vi "GetInvaderBlockEdges.vi"(11 "InvaderPosArray":T2) -> (3 "output cluster":T1)   [LabVIEW 2022 SP3]
uses:
  InvaderPositionArray.ctl
  move_dir_lr.ctl
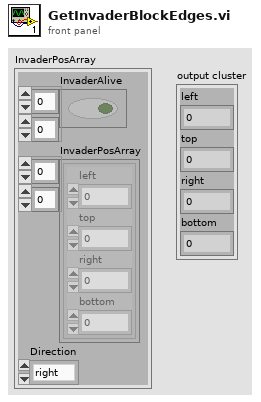
[diagram p1: front panel]
types:
  T1 = cluster{"left":i16, "top":i16, "right":i16, "bottom":i16}
  T2 = typedef "InvaderPositionArray.ctl" = cluster{"InvaderAlive":bool[][], "InvaderPosArray":cluster{"left":i16, "top":i16, "right":i16, "bottom":i16}[][], "Direction":T3}
  T3 = typedef "move_dir_lr.ctl" = enum16{"right", "left"}
  T4 = cluster{"left":i16, "top":i16, "right":i16, "bottom":i16}[][]
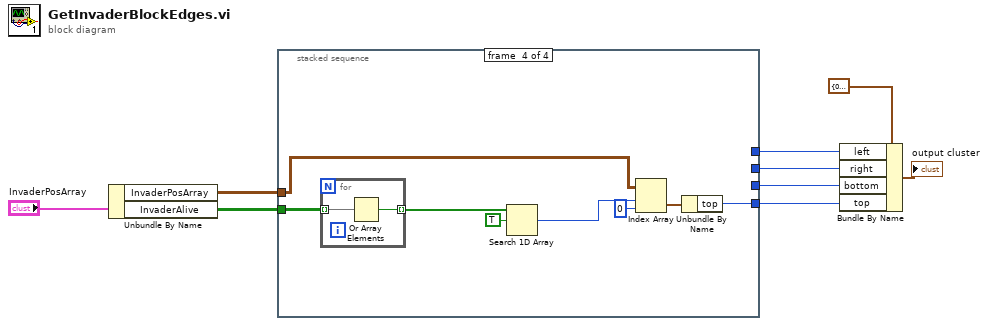
[diagram p0: block diagram]
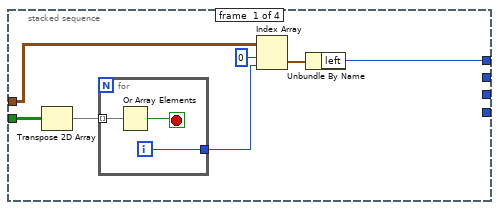
[diagram p2: hidden frame]
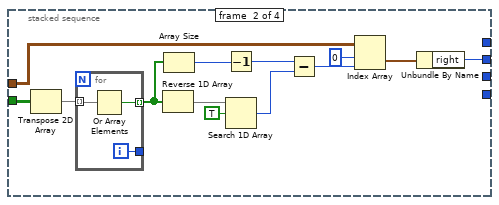
[diagram p3: hidden frame]
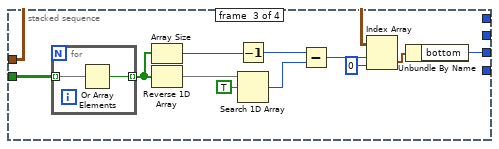
[diagram p4: hidden frame]
diagram:
  n1 = Unbundle By Name("InvaderPosArray") -> ("InvaderPosArray"=w8:T4, "InvaderAlive"=w9:bool[][])
  n2 = stacked-sequence {
    tunnel: w9 -> [w16 w32 w47 w57]
    tunnel: w8 -> [w11 w28 w41 w55]
    tunnel: [w10 _ _ _] -> w6
    tunnel: [_ w25 _ _] -> w5
    tunnel: [_ _ w39 _] -> w4
    tunnel: [_ _ _ w52] -> w2
    frame #0 {
      n3 = Transpose 2D Array(2D array=w16) -> (transposed array=w15:bool[][])
      n4 = for {
        tunnel: w15 -> [w19] mode=indexing
        tunnel: [w17] -> w14
        i -> [w17]
        stop <- w18 stop-if-true
        n5 = Or Array Elements(Boolean array=w19) -> (logical OR=w18:bool)
      }
      n6 = Index Array(array=w11, index (row)=0 ("disabled index (row)"), index (col)=w14) -> (element=w12:T1)
      n7 = Unbundle By Name(w12) -> ("left"=w10:i16)
    }
    frame #1 {
      n8 = Transpose 2D Array(2D array=w32) -> (transposed array=w31:bool[][])
      n9 = for {
        tunnel: w31 -> [w35] mode=indexing
        tunnel: [w34] -> w24 mode=indexing
        tunnel: [w33] -> _
        i -> [w33]
        n10 = Or Array Elements(Boolean array=w35) -> (logical OR=w34:bool)
      }
      n11 = Reverse 1D Array(array=w24) -> (reversed array=w30:bool[])
      n12 = Array Size(array=w24) -> (size(s)=w23:i32)
      n13 = Decrement(x=w23) -> (x-1=w22:i32)
      n14 = Search 1D Array(1D array=w30, element=TRUE) -> (index of element=w21:i32)  [unwired: 1 in]
      n15 = Subtract(x=w22, y=w21) -> (x-y=w20:i32)
      n16 = Index Array(array=w28, index (row)=0 ("disabled index (row)"), index (col)=w20) -> (element=w26:T1)
      n17 = Unbundle By Name(w26) -> ("right"=w25:i16)
    }
    frame #2 {
      n18 = for {
        tunnel: w47 -> [w49] mode=indexing
        tunnel: [w48] -> w40 mode=indexing
        n19 = Or Array Elements(Boolean array=w49) -> (logical OR=w48:bool)
      }
      n20 = Array Size(array=w40) -> (size(s)=w45:i32)
      n21 = Reverse 1D Array(array=w40) -> (reversed array=w42:bool[])
      n22 = Decrement(x=w45) -> (x-1=w44:i32)
      n23 = Search 1D Array(1D array=w42, element=TRUE) -> (index of element=w43:i32)  [unwired: 1 in]
      n24 = Subtract(x=w44, y=w43) -> (x-y=w38:i32)
      n25 = Index Array(array=w41, index (row)=w38, index (col)=0 ("disabled index (col)")) -> (element=w37:T1)
      n26 = Unbundle By Name(w37) -> ("bottom"=w39:i16)
    }
    frame #3 {
      n27 = for {
        tunnel: w57 -> [w59] mode=indexing
        tunnel: [w58] -> w51 mode=indexing
        n28 = Or Array Elements(Boolean array=w59) -> (logical OR=w58:bool)
      }
      n29 = Search 1D Array(1D array=w51, element=TRUE) -> (index of element=w50:i32)  [unwired: 1 in]
      n30 = Index Array(array=w55, index (row)=w50, index (col)=0 ("disabled index (col)")) -> (element=w54:T1)
      n31 = Unbundle By Name(w54) -> ("top"=w52:i16)
    }
  }
  n32 = Bundle By Name(cluster=T1 {"left"=0, "top"=0, "right"=0, "bottom"=0} ("Rectangle"), "left"=w6, "right"=w5, "bottom"=w4, "top"=w2) -> (→"output cluster":T1)
